vi "Check Blacklist.vi"(8 "error in (no error)":errorcluster, 9 "Channel 2":string, 10 "Channel 1":string, 11 "SLSC Switch in":refnum<class "SLSC Switch.lvclass">) -> (0 "error out":errorcluster, 2 "isBlacklisted?":bool, 3 "SLSC Switch out":refnum<class "SLSC Switch.lvclass">)   [LabVIEW 2015, in "SLSC Switch.lvclass"]
uses:
  SLSC Switch.lvclass
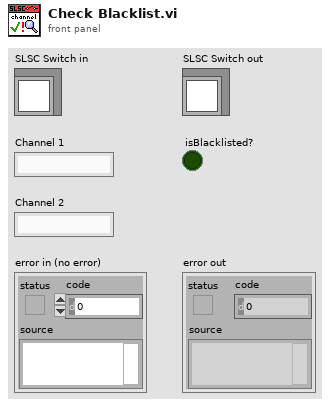
[diagram p1: front panel]
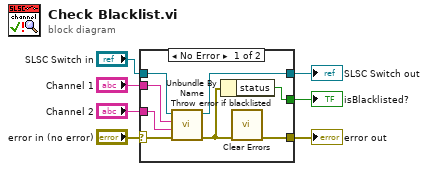
[diagram p0: block diagram]
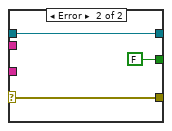
[diagram p2: hidden frame]
diagram:
  n1 = case shown="No Error" "error in (no error)" {
    selector: "error in (no error)" -> [w11 w18]
    tunnel: [w10 w18] -> w6
    tunnel: [w14 w17] -> w4
    tunnel: "SLSC Switch in" -> [w15 w17]
    tunnel: "Channel 1" -> [w13 _]
    tunnel: "Channel 2" -> [w12 _]
    tunnel: [w8 FALSE ("status")] -> w1
    frame No Error {
      n2 = call "Throw error if blacklisted.vi"("error in (no error)"=w11, "Channel 2"=w12, "Channel 1"=w13, "SLSC Switch in"=w15) -> ("error out"=w9:errorcluster, "SLSC Switch out"=w14:refnum<class "SLSC Switch.lvclass">)  [unwired: 5 in, 1 out]
      n3 = Unbundle By Name(w9) -> ("status"=w8:bool)
      n4 = call <vilib>:"Clear Errors.vi"("error in (no error)"=w9) -> ("error out"=w10:errorcluster)  [unwired: 5 in, 1 out]
    }
    frame Error {
    }
  }
  "error out" <- w6
  "SLSC Switch out" <- w4
  "isBlacklisted?" <- w1
